vi "Example Polymorphic 1.vi"   [LabVIEW 2014]
uses:
  just VIs no Translator/Polymorphic Add 2.vi
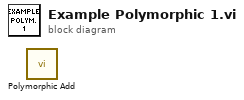
[diagram p0: block diagram]
diagram:
  n1 = call-poly "Polymorphic Add.vi"() -> ()  [unwired: 10 in, 2 out]
